vi "set advance signal.vi"(8 "error in (no error)":errorcluster, 11 "Ixon_Ultra in":refnum<class "Ixon_Ultra.lvclass">) -> (0 "error out":errorcluster, 3 "Ixon_Ultra out":refnum<class "Ixon_Ultra.lvclass">)   [LabVIEW 2018, in "Ixon_Ultra.lvclass"]
uses:
  Ixon_Ultra.lvclass
  C:/Users/Denis/Desktop/S4ACS/S4ACS/Sim_Ixon_Ultra/Sim_Ixon_Ultra.lvclass
  Sim_Ixon_Ultra/Sim_Ixon_Ultra.lvclass/Sim_Ixon_Ultra.ctl
  Sim_Ixon_Ultra/Sim_Ixon_Ultra.lvclass
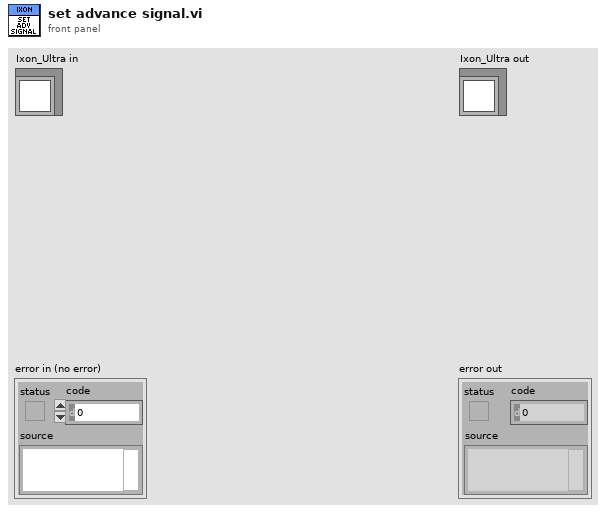
[diagram p1: front panel]
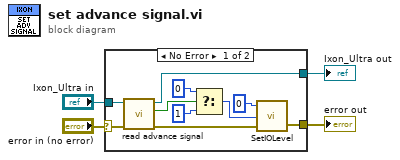
[diagram p0: block diagram]
diagram:
  n1 = case shown="No Error" "error in (no error)" {
    selector: "error in (no error)" -> [w13 w16]
    tunnel: [w11 w16] -> w3
    tunnel: "Ixon_Ultra in" -> [w14 w15]
    tunnel: [w10 w15] -> w1
    frame No Error {
      n2 = call "read advance signal.vi"("error in (no error)"=w13, "Sim_Ixon_Ultra in"=w14) -> ("error out"=w12:errorcluster, "advance signal"=w8:bool, "Sim_Ixon_Ultra out"=w10:refnum<class "Ixon_Ultra.lvclass">)  [unwired: 7 in]
      n3 = Select(t=0, s=w8, f=1) -> (s? t:f=w5:i32)
      n4 = call <userlib>:"SetIOLevel.vi"("error in (no error)"=w12, "Level"=w5, "index"=0) -> ("error out"=w11:errorcluster)  [unwired: 1 out]
    }
    frame Error {
    }
  }
  "error out" <- w3
  "Ixon_Ultra out" <- w1
